vi "Get COM Descriptor.vi"(8 "error in (no error)":errorcluster, 10 "Generate error if no COM port found? (False)":bool, 11 "COM name":string) -> (0 "error out":errorcluster, 2 "COM port Descriptor":string, 3 "COM port":T1)   [LabVIEW 2020, in "Get COM Descriptor.lvlib"]
doc: "Get COM port descriptor string."
uses:
  Get COM Descriptor.lvlib
  COM port.ctl
  <vilib>/Utility/error.llb/Error Cluster From Error Code.vi
  <vilib>/ErrorRing/Error Ring.xnode
  get_com_descriptor.dll
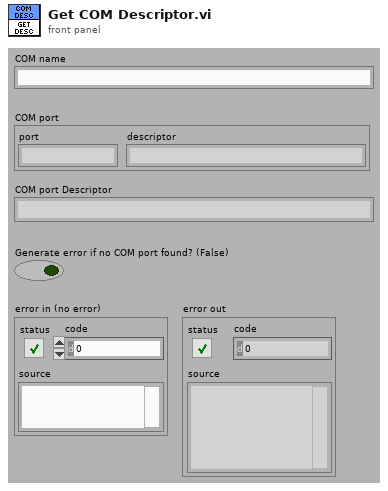
[diagram p1: front panel]
types:
  T1 = typedef "Get COM Descriptor.lvlib/COM port.ctl" = cluster{"port":string, "descriptor":string}
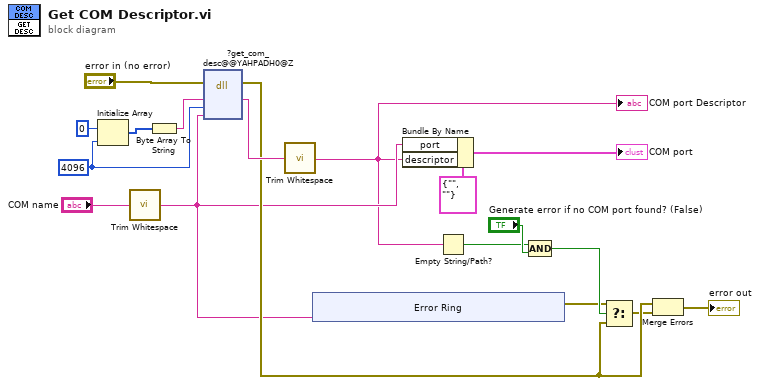
[diagram p0: block diagram]
diagram:
  w14 = 4096 ("dimension size")
  n1 = Initialize Array(u8 0 ("element"), w14) -> (w17:u8[])
  n2 = call <vilib>:"Trim Whitespace.vi"("string"="COM name") -> ("trimmed string"=w4:string)  [unwired: 1 in]
  n3 = Byte Array To String(unsigned byte array=w17) -> (string=w15:string)
  n4 = dll-call lib="F:/Z_bridge_v4/other/get_com_descriptor/get_com_descriptor.dll" fn="?get_com_desc@@YAHPADH0@Z"(error in="error in (no error)", "buf"=w15, "size"=w14, "name"=w4) -> (error out=w8:errorcluster, "buf"=w13:string)  [unwired: 5 in, 1 out]
  n5 = call <vilib>:"Trim Whitespace.vi"("string"=w13) -> ("trimmed string"=w2:string)  [unwired: 1 in]
  "COM port Descriptor" <- w2
  n6 = xnode "Error Ring"("parameter 0"=w4) -> ("error out"=w9:errorcluster)
  n7 = Bundle By Name(cluster=T1 {"port"="", "descriptor"=""} ("COM port"), "port"=w4, "descriptor"=w2) -> (→"COM port":T1)
  n8 = Empty String/Path?(string/path=w2) -> (empty?=w1:bool)
  n9 = Compound Arithmetic op=AND(w1, "Generate error if no COM port found? (False)") -> (w10:bool)
  n10 = Select(t=w9, s=w10, f=w8) -> (s? t:f=w7:errorcluster)
  n11 = Merge Errors(w8, w7) -> (→"error out":errorcluster)
